vi "testMaxFileSize (db - not exceeded).vi"(8 "error in (no error)":errorcluster, 11 "TestCase in":refnum<class "Test-File IO.lvclass">=refnum) -> (0 "error out":errorcluster, 3 "TestCase out":refnum<class "Test-File IO.lvclass">)   [LabVIEW 2019, in "Test-File IO.lvclass"]
uses:
  Test-File IO.lvclass
  Log/Event Level.ctl
  TSC Event Logger.lvlib
  Log/Log.lvclass
  9400858f-8242-4f0f-a3a8-0c5d1ac263e7.vi
  Log Sinks/SQLite Database/SQLite Database.lvclass
  C:/Development/Open Source/tsc-event-logger/Log Sinks/Log Sinks.lvclass
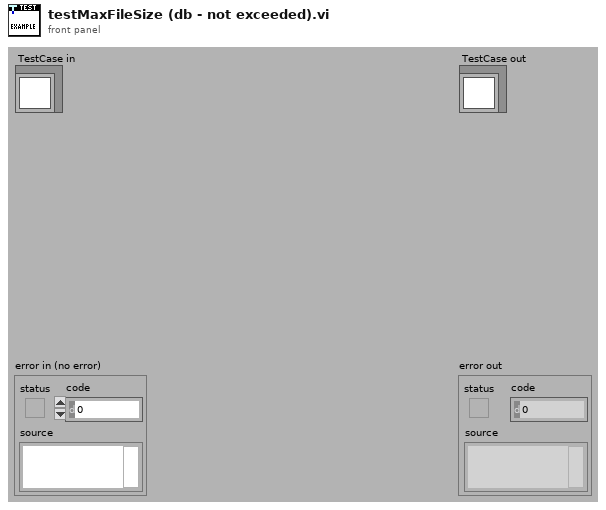
[diagram p1: front panel]
types:
  T1 = typedef "TSC Event Logger.lvlib/Event Level.ctl" = enum16{"OFF", "TRACE", "DEBUG", "INFO", "WARN", "ERROR", "FATAL"}
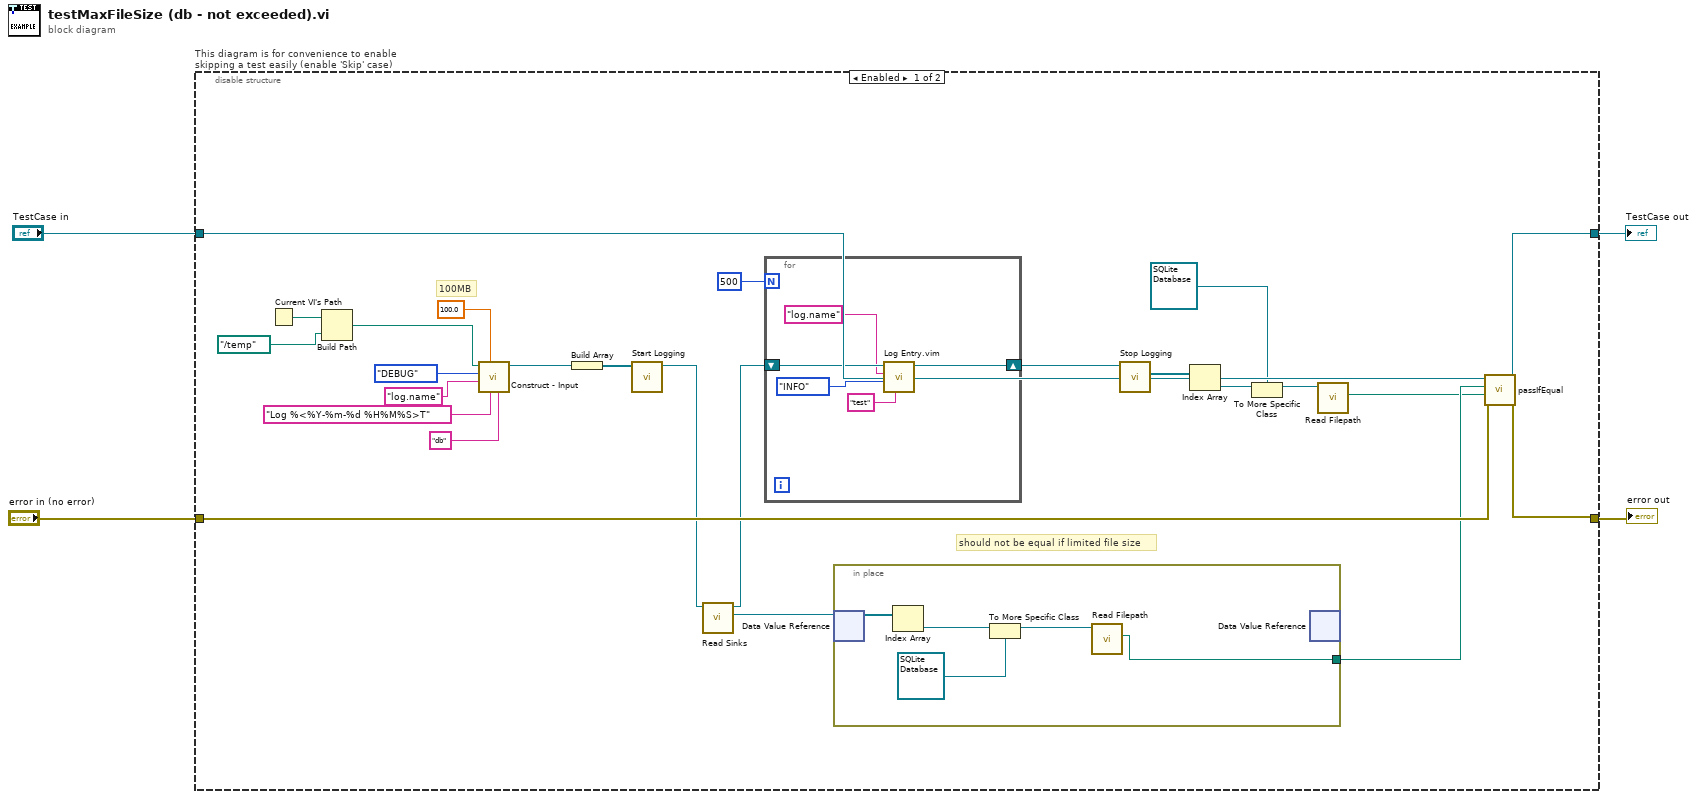
[diagram p0: block diagram]
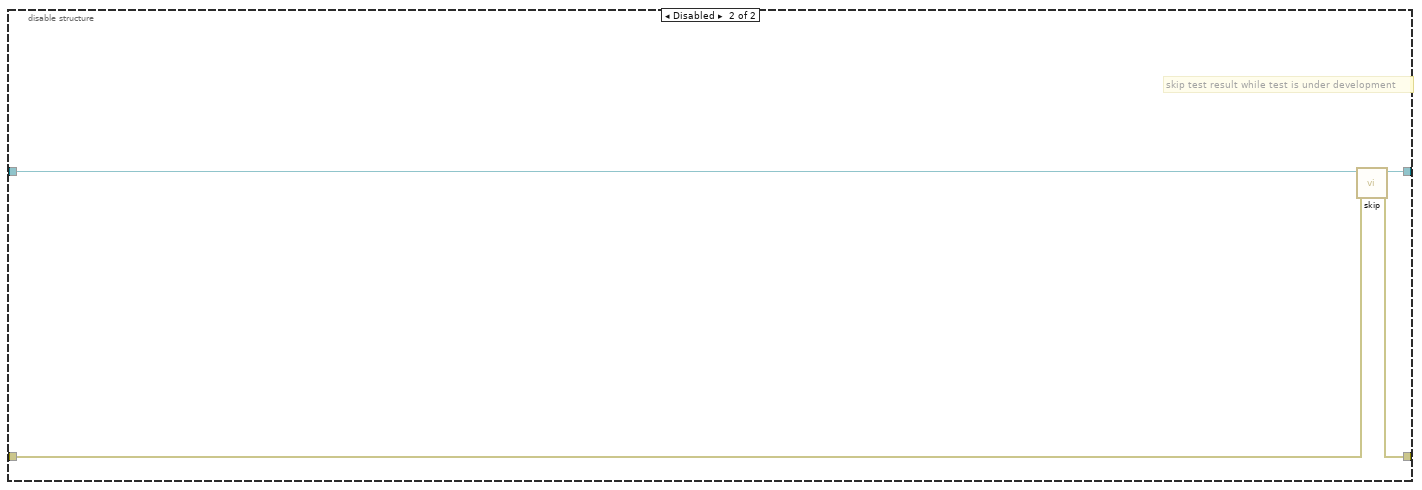
[diagram p2: hidden frame]
diagram:
  n1 = disable-structure "This diagram is for convenience to enable skipping a test easily (enable 'Skip' case)" shown="Enabled" {
    disable-tunnel: "TestCase in" -> [w26 w43]
    disable-tunnel: [w29 w41] -> w1
    disable-tunnel: [w28 w42] -> w3
    disable-tunnel: "error in (no error)" -> [w27 w40]
    frame Enabled {
      # "100MB"
      # "should not be equal if limited file size"
      n2 = Current VI's Path() -> (path=w14:path)
      n3 = Build Path(base path=w14, name or relative path=path "../temp") -> (appended path=w16:path)
      n4 = call "Construct - Input.vi"("extension"="db", "file name format"="Log %<%Y-%m-%d %H%M%S>T", "Max File Size (MB)"=100.0, "Name"="log.name", "Level"=Event_Level."DEBUG", "log location"=w16) -> ("SQLite Database out"=w9:refnum<class "SQLite Database.lvclass">)  [unwired: 4 in, 1 out]
      n5 = Build Array(w9) -> (w8:refnum<class "SQLite Database.lvclass">[])
      n6 = call "Start Logging.vi"("Sinks"=w8) -> ("Logger"=w6:refnum<class "Log.lvclass">)  [unwired: 9 in, 1 out]
      n7 = call "Read Sinks.vi"("Log in"=w6) -> ("Sink DVR Array"=w25:refnum<data-value>, "Log out"=w20:refnum<class "Log.lvclass">)  [unwired: 9 in]
      n8 = for {
        N: 500 -> [_]
        shift-right: [w37] -> w21
        shift-left: w20 -> [w38]
        n9 = call "Log Entry.vim"("Message"="test", "Level"=Event_Level."INFO", "Logger"="log.name", "Log in"=w38) -> ("Log out"=w37:refnum<class "Log.lvclass">)  [unwired: 6 in, 1 out]
      }
      n10 = in-place {
        in-place-border: [w30] -> w24
        n11 = in-place-dvr #1(w25) -> (w34:refnum<class "Log Sinks.lvclass">[])  [unwired: 1 out]
        n12 = Index Array(array=w34) -> (element=w33:refnum<class "Log Sinks.lvclass">)  [unwired: 1 in]
        n13 = To More Specific Class(target class=refnum<class "SQLite Database.lvclass"> refnum ("TSC Event Logger.lvlib:SQLite Database.lvclass"), reference=w33) -> (specific class reference=w32:refnum<class "SQLite Database.lvclass">)  [unwired: 1 in, 1 out]
        n14 = call "Read Filepath.vi"("SQLite Database in"=w32) -> ("File Path Indicator"=w30:path)  [unwired: 9 in, 1 out]
        n15 = in-place-dvr #1() -> ()  [unwired: 1 in, 2 out]
      }
      n16 = call "Stop Logging.vi"("Logger"=w21) -> ("sinks"=w17:refnum<class "Log Sinks.lvclass">[])  [unwired: 9 in, 1 out]
      n17 = Index Array(array=w17) -> (element=w19:refnum<class "Log Sinks.lvclass">)  [unwired: 1 in]
      n18 = To More Specific Class(target class=refnum<class "SQLite Database.lvclass"> refnum ("TSC Event Logger.lvlib:SQLite Database.lvclass"), reference=w19) -> (specific class reference=w18:refnum<class "SQLite Database.lvclass">)  [unwired: 1 in, 1 out]
      n19 = call "Read Filepath.vi"("SQLite Database in"=w18) -> ("File Path Indicator"=w22:path)  [unwired: 9 in, 1 out]
      n20 = call-dynamic "passIfEqual.vi"("error in (no error)"=w27, "y"=w22, "x"=w24, "TestCase in"=w26) -> ("error out"=w28:errorcluster, "TestCase out"=w29:refnum<class "Test-File IO.lvclass">)  [unwired: 6 in]
    }
    frame Disabled {
      # "skip test result while test is under development"
      n21 = call <vilib>:"skip.vi"("error in (no error)"=w40, "TestCase in"=w43) -> ("error out"=w42:errorcluster, "TestCase out"=w41:refnum<class "Test-File IO.lvclass">)  [unwired: 8 in]
    }
  }
  "error out" <- w3
  "TestCase out" <- w1
